vi "ICM aU16.vi"(9 "Reverse Bytes":bool, 11 "String In":string) -> (1 "Value U16":u16, 2 "Value":dbl, 3 "String Out":string)   [LabVIEW 2024]
doc: "ICM aU16.vi\n\n This VI is used to parse binary data that contains a U16 integer.\n\nThis VI was original part of the OSDS system.\n\nInstrument Communication Module Version 1.0\nSeptember, 2017 Original Code Consulting David Thomson\n www.originalcode.com"
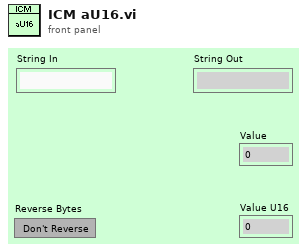
[diagram p1: front panel]
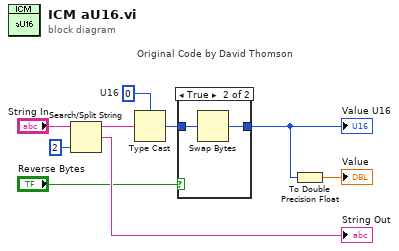
[diagram p0: block diagram]
diagram:
  w7 = u16 0  # U16
  n1 = Search/Split String(string="String In", offset (0)=2) -> (substring before match=w2:string, match + rest of string=→"String Out":string)  [unwired: 2 out]
  n2 = Type Cast(type=w7, x=w2) -> (*(type *) &x=w3:u16)
  n3 = case "Original Code by David Thomson" shown="True" "Reverse Bytes" {
    tunnel: w3 -> [w10 w12]
    tunnel: [w10 w11] -> w1
    frame False {
    }
    frame True {
      n4 = Swap Bytes(anything=w12) -> (byte swapped=w11:u16)
    }
  }
  "Value U16" <- w1
  n5 = To Double Precision Float(number=w1) -> (double precision float=→"Value":dbl)
